vi "Finite Potential Well.vi"() -> ()   [LabVIEW 2023]
doc: "This VI shows how to solve Schrodinger's equation for when a particle is trapped in a finite potential well."
panel:
  in  "Stop":bool
  in  "m [kg]":dbl=9.11e-31
  in  "L [nm]":dbl(slide)=2.0 scale=1e-06..2.0
  in  "V0 [eV]":dbl(slide)=10.000000000000002 scale=10.0..10000.0
  in  "Quantum Number":i32(slide)=1 scale=1.0..100.0
  out "Wave Function":cluster{"x":dbl[], "y":dbl[]}(graph)
  out "Probability Density":cluster{"x":dbl[], "y":dbl[]}(graph)
  out "E [eV]":dbl
  # "Overview: Demonstrates how to use the MATLAB Node and MATLAB(R) to solve Schrodinger's equation describing a particle trapped in a finite potential well.\nRequirements: LabVIEW Full Development System, MATLAB(R) Application Software release R2016a or later. \nInstructions:\n1. Run this VI.\n2. Change the V0 and Quantum Number parameters. Observe the output Wave Function and Probability Density, especially in the region beyond the -L to L range marked by red cursor.\n3. Click Stop to stop the VI."
  # "Finite Potential Well"
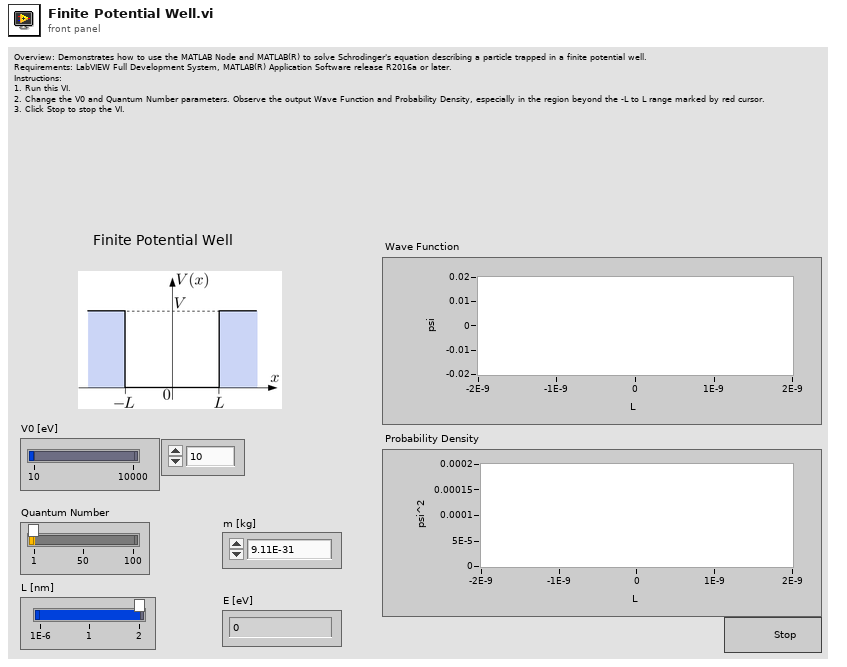
[diagram p1: front panel]
types:
  T1 = cluster{"E [eV]":dbl, "Wave Function":cluster{"x":dbl[], "y":dbl[]}, "Probability Density":cluster{"x":dbl[], "y":dbl[]}}
  T2 = cluster{"R":dbl, "L":dbl, "hbar":dbl, "V0":dbl, "m":dbl}
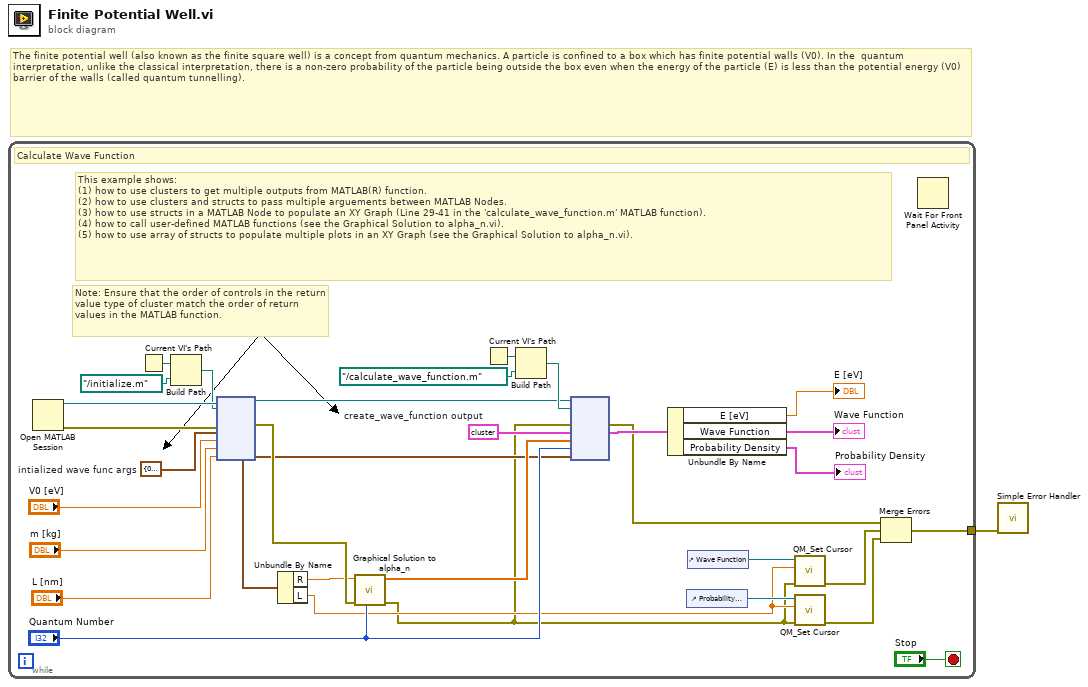
[diagram p0: block diagram]
diagram:
  # "The finite potential well (also known as the finite square well) is a concept from quantum mechanics. A particle is confined to a box which has finite potential walls (V0). In the  quantum interpretation, unlike the classical interpretation, there is a non-zero probability of the particle being outside the box even when the energy of the particle (E) is less than the potential energy (V0) barrier of the walls (called quantum tunnelling)."
  n1 = while {
    tunnel: [w29] -> w1
    stop <- "Stop" stop-if-true
    w14 = T1 {"E [eV]"=0.0, "Wave Function"={"x"=array[30003 elements], "y"=array[30003 elements]}, "Probability Density"={"x"=array[30003 elements], "y"=array[30003 elements]}}  # create_wave_function output
    w22 = T2 {"R"=0.0, "L"=0.0, "hbar"=0.0, "V0"=0.0, "m"=0.0}  # intialized wave func args
    # "Note: Ensure that the order of controls in the return value type of cluster match the order of return values in the MATLAB function."
    # "This example shows:\n(1) how to use clusters to get multiple outputs from MATLAB(R) function.\n(2) how to use clusters and structs to pass multiple arguements between MATLAB Nodes.\n(3) how to use structs in a MATLAB Node to populate an XY Graph (Line 29-41 in the 'calculate_wave_function.m' MATLAB function).\n(4) how to call user-defined MATLAB functions (see the Graphical Solution to alpha_n.vi).\n(5) how to use array of structs to populate multiple plots in an XY Graph (see the Graphical Solution to alpha_n.vi)."
    # "Calculate Wave Function"
    n2 = Open MATLAB Session() -> (8:w27:refnum<k37>, 11:w26:errorcluster)  [unwired: 2 in]
    n3 = Current VI's Path() -> (path=w25:path)
    n4 = Build Path(base path=w25, name or relative path=path "../initialize.m") -> (appended path=w23:path)
    n5 = node(w27, w23, w26, w22, "V0 [eV]", "m [kg]", "L [nm]") -> (w15:refnum<k37>, w11:errorcluster, w3:T2)  [unwired: 4 in, 2 out]
    n6 = Unbundle By Name(w3) -> ("R"=w9:dbl, "L"=w8:dbl)
    n7 = call "Graphical Solution to alpha_n.vi"("Quantum Number"="Quantum Number", "error in"=w11, "R"=w9) -> ("error out"=w2:errorcluster, "alpha_n"=w13:dbl[])  [unwired: 6 in, 1 out]
    n8 = Current VI's Path() -> (path=w17:path)
    n9 = Build Path(base path=w17, name or relative path=path "../calculate_wave_function.m") -> (appended path=w16:path)
    n10 = node(w15, w16, w2, w14, w13, "Quantum Number", w3) -> (w4:errorcluster, w12:T1)  [unwired: 4 in, 3 out]
    n11 = Unbundle By Name(w12) -> ("E [eV]"=→"E [eV]":dbl, "Wave Function"=→"Wave Function":cluster{"x":dbl[], "y":dbl[]}, "Probability Density"=→"Probability Density":cluster{"x":dbl[], "y":dbl[]})
    n12 = control-ref of="Probability Density"() -> (w32:refnum<vi>)
    n13 = control-ref of="Wave Function"() -> (w33:refnum<vi>)
    n14 = call "QM_Set Cursor.vi"("error in (no error)"=w2, "L"=w8, "XYGraph in"=w33) -> ("error out"=w31:errorcluster)  [unwired: 8 in]
    n15 = call "QM_Set Cursor.vi"("error in (no error)"=w2, "L"=w8, "XYGraph in"=w32) -> ("error out"=w30:errorcluster)  [unwired: 8 in]
    n16 = Merge Errors(w4, w31, w30) -> (w29:errorcluster)
    n17 = Wait For Front Panel Activity() -> ()  [unwired: 3 in, 1 out]
  }
  n18 = call <vilib>:"Simple Error Handler.vi"("error in (no error)"=w1) -> ()  [unwired: 4 in, 5 out]
